vi "AOL Z Cal-Init.vi"(8 "error in (no error)":errorcluster, 11 "Pre-AOL Z wizard refs":T2) -> (0 "error out":errorcluster, 2 "Cal settings window's title":string, 3 "Initial state":T1)   [LabVIEW 2017]
uses:
  Typedefs/Pre-AOL Z wizard refs.ctl
  Typedefs/Cal mode.ctl
  Typedefs/AOL Z cal wizard states.ctl
  Globals/gl_Calibration globals.vi
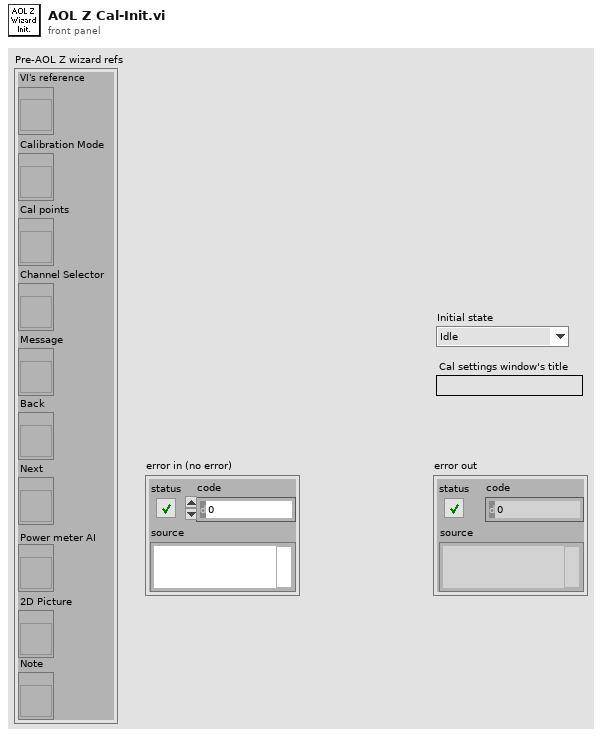
[diagram p1: front panel]
types:
  T1 = typedef "AOL Z cal wizard states.ctl" = enum16{"Idle", "Select cal mode", "Select cal points", "Select channel", "Start calibration"}
  T2 = typedef "Pre-AOL Z wizard refs.ctl" = cluster{"VI's reference":refnum<vi>, "Calibration Mode":refnum<vi>, "Cal points":refnum<vi>, "Channel Selector":refnum<vi>, "Message":refnum<vi>, "Back":refnum<vi>, "Next":refnum<vi>, "Power meter AI":refnum<vi>, "2D Picture":refnum<vi>, "Note":refnum<vi>}
  T3 = typedef "Cal mode.ctl" = enum16{"Automatic", "Interactive"}
  T4 = enum8{"Enabled", "Disabled", "Disabled and Grayed Out"}
  T5 = typedef "Cal points.ctl" = enum16{"5-points calibration (crude)", "11-points calibration", "21-points calibration", "41-points calibration"}
  T6 = typedef "Cal channel.ctl" = enum16{"Red Channel", "Green Channel"}
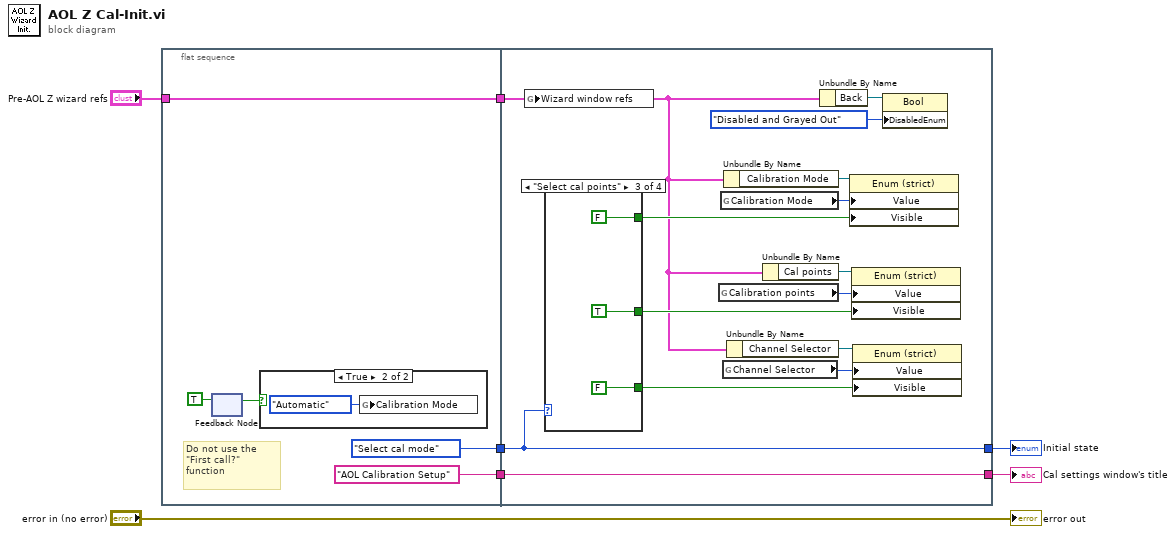
[diagram p0: block diagram]
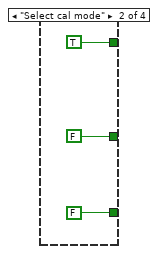
[diagram p4: hidden frame]
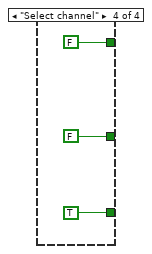
[diagram p5: hidden frame]
diagram:
  n1 = flat-sequence {
    tunnel: "Pre-AOL Z wizard refs" -> [w12]
    tunnel: [w12] -> w3
    tunnel: [AOL_Z_cal_wizard_states."Select cal mode" ("Initial state")] -> w2
    tunnel: ["AOL Calibration Setup"] -> w1
    tunnel: [w15] -> w5
    tunnel: [w14] -> w4
    tunnel: w3 -> [w17]
    tunnel: w2 -> [w15]
    tunnel: w1 -> [w14]
    frame #0 {
      # "Do not use the \"First call?\" function"
      n2 = feedback #1() -> (w11:bool)  [unwired: 1 in]
      n3 = feedback-in #1(TRUE) -> ()
      n4 = case shown="True" w11 {
        frame False {
        }
        frame True {
          n5 = global write "gl_Calibration globals.vi" "Calibration Mode"(Cal_mode."Automatic" ("Calibration Mode")) -> ()
        }
      }
    }
    frame #1 {
      n6 = global write "gl_Calibration globals.vi" "Wizard window refs"(w17) -> ()
      n7 = case shown="\"Select cal points\"" w15 {
        tunnel: [_ FALSE ("Visible") TRUE ("Visible") FALSE ("Visible")] -> w27
        tunnel: [_ FALSE ("Visible") FALSE ("Visible") TRUE ("Visible")] -> w26
        tunnel: [_ TRUE ("Visible") FALSE ("Visible") FALSE ("Visible")] -> w25
        frame "Idle", Default {
        }
        frame "Select cal mode" {
        }
        frame "Select cal points" {
        }
        frame "Select channel" {
        }
      }
      n8 = global read "gl_Calibration globals.vi" "Calibration points"() -> (w23:T5)
      n9 = global read "gl_Calibration globals.vi" "Calibration Mode"() -> (w22:T3)
      n10 = global read "gl_Calibration globals.vi" "Channel Selector"() -> (w24:T6)
      n11 = Unbundle By Name(w17) -> ("Calibration Mode"=w19:refnum<vi>)
      n12 = Unbundle By Name(w17) -> ("Channel Selector"=w21:refnum<vi>)
      n13 = Unbundle By Name(w17) -> ("Cal points"=w20:refnum<vi>)
      n14 = Unbundle By Name(w17) -> ("Back"=w18:refnum<vi>)
      n15 = property on="Property Node" class="Enum (strict)"(reference=w19, "Value"=w22, "Visible"=w25) -> ()  [unwired: 1 in, 2 out]
      n16 = property on="Property Node" class="Enum (strict)"(reference=w20, "Value"=w23, "Visible"=w27) -> ()  [unwired: 1 in, 2 out]
      n17 = property on="Property Node" class="Enum (strict)"(reference=w21, "Value"=w24, "Visible"=w26) -> ()  [unwired: 1 in, 2 out]
      n18 = property on="Property Node" class="Bool"(reference=w18, "DisabledEnum"=T4."Disabled and Grayed Out" ("Disabled")) -> ()  [unwired: 1 in, 2 out]
    }
  }
  "error out" <- "error in (no error)"
  "Initial state" <- w5
  "Cal settings window's title" <- w4
